vi "PH_Synchrolock_Watch.PC Set Limit.vi"(0 "i ref in":refnum<vi>, 1 "Limit to set":T1 items=["Mean Phase upper Limit", "Mean Phase lower Limit", "RF Amplutude lower Limit", "Mira Amplidute upper Limit", "Mira Amplidute lower Limit"], 2 "Limit":dbl=100.0, 5 "error in":errorcluster) -> (14 "i ref out":refnum<vi>, 19 "error out":errorcluster)   [LabVIEW 2014, in "PH_Synchrolock_Watch.lvlib"]
doc: "This VI writes incoming information to own attributes and sets the hardware."
uses:
  PH_Synchrolock_Watch.lvlib
  PH_Synchrolock_Watch.Limit to set.ctl
  PH_Basics/PH_Common/PH_Common.lvlib
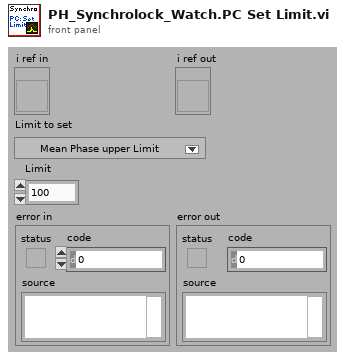
[diagram p1: front panel]
types:
  T1 = typedef "PH_Synchrolock_Watch.lvlib/PH_Synchrolock_Watch.Limit to set.ctl" = i16
  T2 = typedef "PH_Synchrolock_Watch.lvlib/PH_Synchrolock_Watch.i attribute.ctl" = cluster{"GUI Refs":cluster{"Mean Phase Graph":refnum<vi>, "RF Amplitude Graph":refnum<vi>, "Mira Amplitude Graph":refnum<vi>, "MIRA State":refnum<vi>, "Mean Phase":refnum<vi>, "RF Amplitude":refnum<vi>, "Mira Amplitude":refnum<vi>, "Mean Phase in range?":refnum<vi>, "RF Amplitude above limit?":refnum<vi>, "Mira Amplitude in range?":refnum<vi>, "Mean phase upper limit":refnum<vi>, "Mean phase lower limit":refnum<vi>, "RF Amplitude lower limit":refnum<vi>, "Mira Amplitude lower limit":refnum<vi>, "Mira Amplitude upper limit":refnum<vi>, "Mira scope":refnum<vi>, "Reset Mira warning":refnum<vi>}, "Status":cluster{"Reset Warning":bool}, "Mean Phase":cluster{"Current Value":dbl, "Upper Limit":dbl, "Lower Limit":dbl, "Data":cluster{dbl[], dbl[]}}, "RF":cluster{"Current Value":dbl, "Lower Limit":dbl, "Data":cluster{dbl[], dbl[]}}, "MIRA":cluster{"Current Value":dbl, "Upper Limit":dbl, "Lower Limit":dbl, "Data":cluster{dbl[], dbl[]}}}
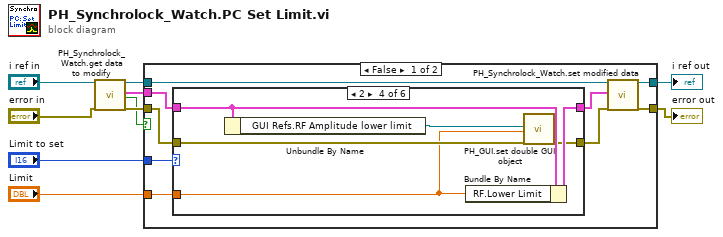
[diagram p0: block diagram]
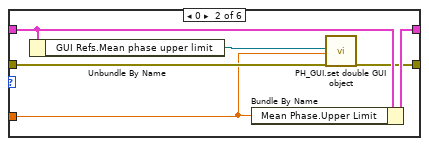
[diagram p3: hidden frame]
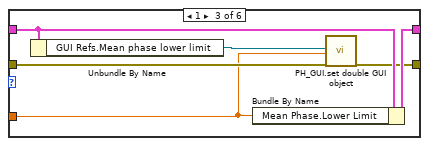
[diagram p4: hidden frame]
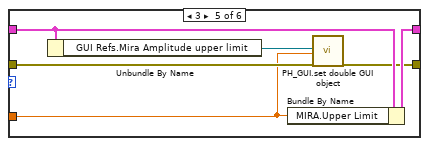
[diagram p5: hidden frame]
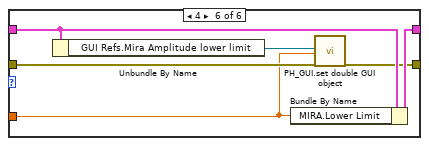
[diagram p6: hidden frame]
diagram:
  n1 = call "PH_Synchrolock_Watch.get data to modify.vi"("i ref in"="i ref in", "error in (no error)"="error in") -> ("i ref out"=w7:refnum<vi>, "i attribute"=w1:T2, "timed out"=w2:bool, "error out"=w8:errorcluster)  [unwired: 14 in]
  n2 = case shown="False" w2 {
    tunnel: w8 -> [w14 w52]
    tunnel: [w17 w53] -> w6
    tunnel: [w19 w52] -> w5
    tunnel: w7 -> [w18 w53]
    tunnel: "Limit" -> [w12 _]
    tunnel: "Limit to set" -> [w11 _]
    tunnel: w1 -> [w15 _]
    frame False {
      n3 = case shown="2" w11 {
        tunnel: [w20 w27 w33 w39 w45 w51] -> w16
        tunnel: w15 -> [w20 w26 w32 w38 w44 w50]
        tunnel: w14 -> [w21 w24 w30 w36 w42 w48]
        tunnel: [w21 w23 w29 w35 w41 w47] -> w13
        tunnel: w12 -> [_ w22 w28 w34 w40 w46]
        frame Default {
        }
        frame 0 {
          n4 = Unbundle By Name(w26) -> ("GUI Refs.Mean phase upper limit"=w25:refnum<vi>)
          n5 = Bundle By Name(cluster=w26, "Mean Phase.Upper Limit"=w22) -> (w27:T2)
          n6 = call "PH_GUI.set double GUI object.vi"("GUI object Ref"=w25, "value"=w22, "error in (no error)"=w24) -> ("error out"=w23:errorcluster)  [unwired: 16 in]
        }
        frame 1 {
          n7 = Unbundle By Name(w32) -> ("GUI Refs.Mean phase lower limit"=w31:refnum<vi>)
          n8 = Bundle By Name(cluster=w32, "Mean Phase.Lower Limit"=w28) -> (w33:T2)
          n9 = call "PH_GUI.set double GUI object.vi"("GUI object Ref"=w31, "value"=w28, "error in (no error)"=w30) -> ("error out"=w29:errorcluster)  [unwired: 16 in]
        }
        frame 2 {
          n10 = Unbundle By Name(w38) -> ("GUI Refs.RF Amplitude lower limit"=w37:refnum<vi>)
          n11 = Bundle By Name(cluster=w38, "RF.Lower Limit"=w34) -> (w39:T2)
          n12 = call "PH_GUI.set double GUI object.vi"("GUI object Ref"=w37, "value"=w34, "error in (no error)"=w36) -> ("error out"=w35:errorcluster)  [unwired: 16 in]
        }
        frame 3 {
          n13 = Unbundle By Name(w44) -> ("GUI Refs.Mira Amplitude upper limit"=w43:refnum<vi>)
          n14 = Bundle By Name(cluster=w44, "MIRA.Upper Limit"=w40) -> (w45:T2)
          n15 = call "PH_GUI.set double GUI object.vi"("GUI object Ref"=w43, "value"=w40, "error in (no error)"=w42) -> ("error out"=w41:errorcluster)  [unwired: 16 in]
        }
        frame 4 {
          n16 = Unbundle By Name(w50) -> ("GUI Refs.Mira Amplitude lower limit"=w49:refnum<vi>)
          n17 = Bundle By Name(cluster=w50, "MIRA.Lower Limit"=w46) -> (w51:T2)
          n18 = call "PH_GUI.set double GUI object.vi"("GUI object Ref"=w49, "value"=w46, "error in (no error)"=w48) -> ("error out"=w47:errorcluster)  [unwired: 16 in]
        }
      }
      n19 = call "PH_Synchrolock_Watch.set modified data.vi"("i ref in"=w18, "i attribute"=w16, "error in (no error)"=w13) -> ("i ref out"=w17:refnum<vi>, "error out"=w19:errorcluster)  [unwired: 15 in]
    }
    frame True {
    }
  }
  "error out" <- w5
  "i ref out" <- w6
